vi "Get Command Queue.vi"(8 "error in (no error)":errorcluster) -> (0 "error out":errorcluster, 3 "Queue out":refnum<queue>)   [LabVIEW 2016, in "Drive System.lvlib"]
uses:
  Drive System.lvlib
  DriveCmd.ctl
  DriveCmdList.ctl
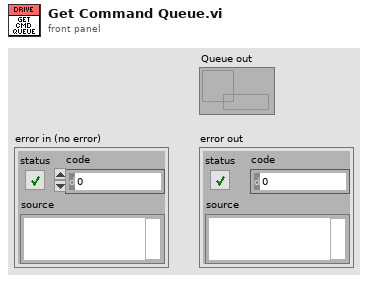
[diagram p1: front panel]
types:
  T1 = typedef "Drive System.lvlib/DriveCmd.ctl" = cluster{"cmd":T2, "data":variant, "Force? (F)":bool, "Lock":string}
  T2 = typedef "Drive System.lvlib/DriveCmdList.ctl" = enum16{"Idle", "Cleanup", "Drive For Time", "Follow Path", "Drive Tank", "Drive Arcade", "Unlock", "Lock"}
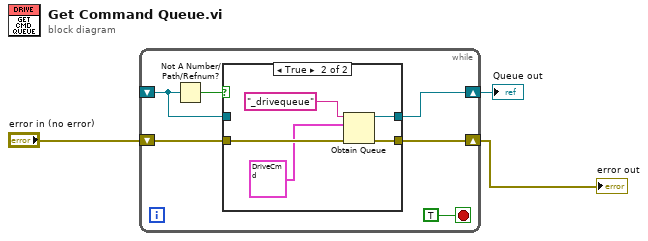
[diagram p0: block diagram]
diagram:
  n1 = while {
    shift-right: [w8] -> w2
    shift-left: "error in (no error)" -> [w9]
    shift-right: [w7] -> w1
    shift-left: _ -> [w5]
    stop <- TRUE stop-if-true
    n2 = Not A Number/Path/Refnum?(number/path/refnum=w5) -> (NaN/Path/Refnum?=w6:bool)
    n3 = case shown="True" w6 {
      tunnel: w9 -> [w10 w16]
      tunnel: [w10 w15] -> w8
      tunnel: [w11 w14] -> w7
      tunnel: w5 -> [w11 _]
      frame False {
      }
      frame True {
        n4 = Obtain Queue(name (unnamed)="_drivequeue", element data type=T1 {"cmd"=enum."Cleanup", "data"=variant, "Force? (F)"=FALSE, "Lock"=""}, error in (no error)=w16) -> (queue out=w14:refnum<queue>, error out=w15:errorcluster)  [unwired: 2 in, 1 out]
      }
    }
  }
  "error out" <- w2
  "Queue out" <- w1
